vi "Enter.vi"(8 "error in (no error)":errorcluster, 11 "Room in":refnum<class "Room.lvclass">) -> (0 "error out":errorcluster, 3 "Room out":refnum<class "Room.lvclass">)   [LabVIEW 2016, in "Room.lvclass"]
uses:
  Room.lvclass
  MapSite/MapSite.lvclass
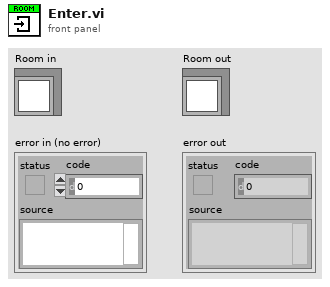
[diagram p1: front panel]
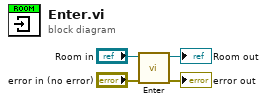
[diagram p0: block diagram]
diagram:
  n1 = call-parent "Enter.vi"("error in (no error)"="error in (no error)", "MapSite in"="Room in") -> ("error out"=→"error out":errorcluster, "MapSite out"=→"Room out":refnum<class "Room.lvclass">)  [unwired: 8 in]
